vi "firma.vi"() -> ()   [LabVIEW 2016]
uses:
  <vilib>/Utility/miscctls.llb/LVMouseTypeDef.ctl
  <vilib>/Analysis/1siggen.llb/Ramp Pattern by Samples.vi
  <vilib>/gmath/NI_Gmath.lvlib
  <vilib>/Analysis/NI_AALBase.lvlib
panel:
  out "Waveform Graph 4":waveform(dbl)(graph)
  out "XY Graph":cluster{i32[], i32[]}(graph)
  out "x":i32[](graph)
  out "y":i32[](graph)
  out "Mouse":T1
  in  "Stop Button":bool
  in  "pen":T2={"Width"=1, "Style"=enum."Solid"}
  out "new picture":picture
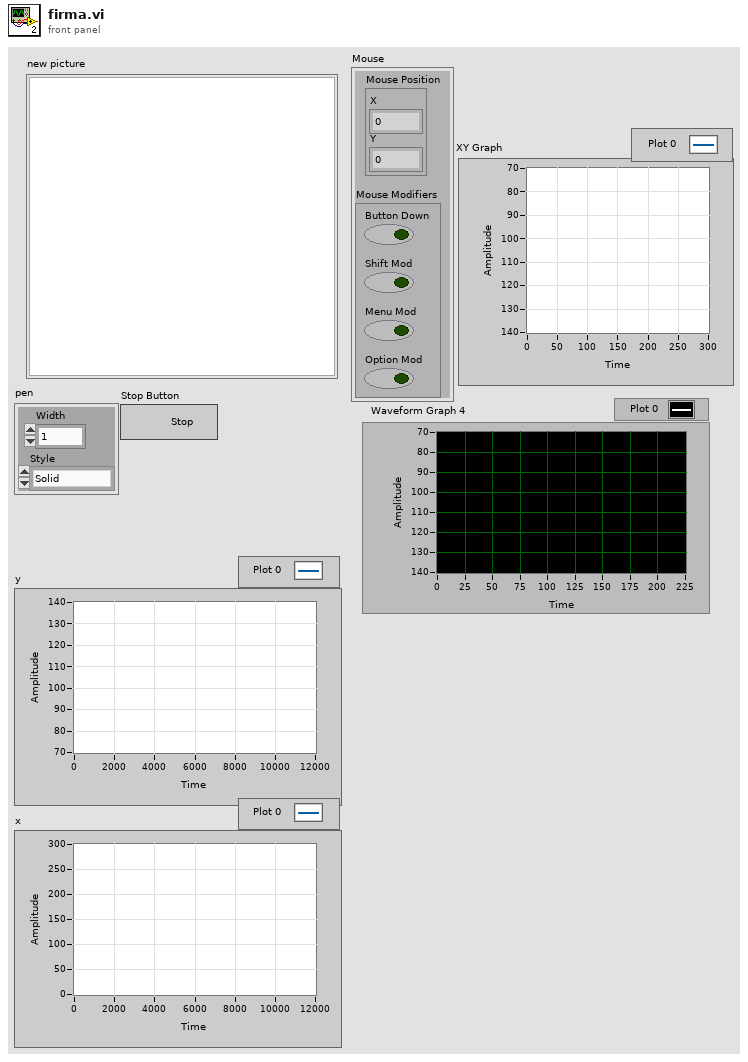
[diagram p1: front panel]
types:
  T1 = typedef "LVMouseTypeDef.ctl" = cluster{"Mouse Position":cluster{"X":i32, "Y":i32}, "Mouse Modifiers":cluster{"Button Down":bool, "Shift Mod":bool, "Menu Mod":bool, "Option Mod":bool}}
  T2 = cluster{"Width":u16, "Style":enum32{"Solid", "Dash", "Dot", "DashDot", "DashDotDot"}}
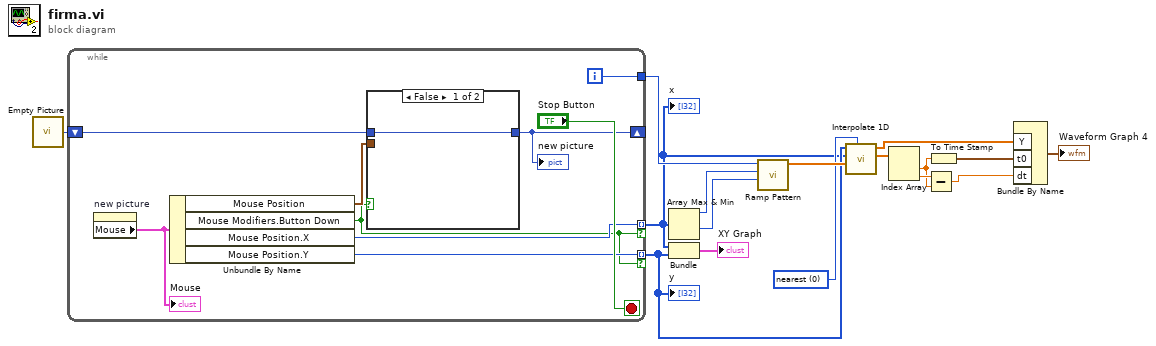
[diagram p0: block diagram]
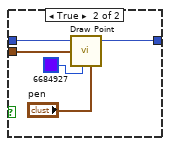
[diagram p2: hidden frame]
diagram:
  w8 = 0 items=["nearest", "linear", "spline", "cubic Hermite", "Lagrange"] ("method")
  n1 = call "Empty Picture"() -> ("empty picture"=w16:picture)
  n2 = while {
    shift-right: [w24] -> _
    shift-left: w16 -> [w23]
    tunnel: [w20] -> w1 mode=indexing if=w18
    tunnel: [w19] -> w2 mode=indexing if=w18
    tunnel: [w17] -> w4
    i -> [w17]
    stop <- "Stop Button" stop-if-true
    n3 = property on="new picture" class="Pict"() -> ("Mouse"=w22:T1)  [unwired: 2 in, 2 out]
    "Mouse" <- w22
    n4 = Unbundle By Name(w22) -> ("Mouse Position"=w21:cluster{"X":i32, "Y":i32}, "Mouse Modifiers.Button Down"=w18:bool, "Mouse Position.X"=w20:i32, "Mouse Position.Y"=w19:i32)
    n5 = case shown="False" w18 {
      tunnel: [w26 w29] -> w24
      tunnel: w23 -> [w26 w28]
      tunnel: w21 -> [_ w27]
      frame False {
      }
      frame True {
        n6 = call <vilib>:"Draw Point.vi"("picture"=w28, "point(x,y)"=w27, "color(black)"=u32 6684927, "pen"="pen") -> ("new picture"=w29:picture)  [unwired: 5 in]
      }
    }
    "new picture" <- w24
  }
  "y" <- w2
  "x" <- w1
  n7 = Array Max & Min(array=w1) -> (max value=w14:i32, min value=w13:i32)  [unwired: 2 out]
  n8 = Bundle(w1, w2) -> (→"XY Graph":cluster{i32[], i32[]})  [unwired: 1 in]
  n9 = call-poly <vilib>:"Ramp Pattern.vi"("start"=w13, "end"=w14, "samples"=w4) -> ("Ramp Pattern"=w10:dbl[])  [unwired: 7 in, 1 out]
  n10 = call <vilib>:"Interpolate 1D.vi"("method"=w8, "xi"=w10, "X"=w1, "Y"=w2) -> ("xi used"=w7:dbl[], "yi"=w9:dbl[])  [unwired: 2 in, 4 out]
  n11 = Index Array(array=w7) -> (element #1=w5:dbl, element #2=w6:dbl)  [unwired: 2 in]
  n12 = Subtract(x=w6, y=w5) -> (x-y=w3:dbl)
  n13 = To Time Stamp(1:w5) -> (0:w12:timestamp)
  n14 = Bundle By Name("Y"=w9, "t0"=w12, "dt"=w3) -> (→"Waveform Graph 4":waveform(dbl))  [unwired: 1 out]
